vi "PV OnTool Operating adjustment.vi"(8 "error in (no error)":errorcluster, 9 "PV OnTool Op adjustment - Cluster":T1={"Parameter"=0, "Parameter\nread only<->describe"=FALSE, "off<->on"=TRUE, "Rotation speed set value\nin rot. speed setting\noperations [%]"=100.0, "Operations mode pump"=0} {"Operations mode pump" items=[" Rotations speed", " Final Speed operation", " Loadlock (Softpumping)", " Idle"]; "Rotation speed set value\nin rot. speed setting\noperations [%]" min=15.0 max=100.0 step=0.1 format="%.2f"; "Parameter" items=[" Pumping station", " Operations mode pump", " Rotation speed set value in rot. speed setting operations", " Set rotation speed BkP [Hz] (read only)", " Actual rotation speed BkP [Hz] (read only)", " Power supply version"]}, 10 "Adress of unit":u16=1 min=1 max=999 step=1, 11 "VISA session":refnum<visa-resource-name>) -> (0 "error out":errorcluster, 2 "response (data)":string, 3 "dup VISA session":refnum<visa-resource-name>)   [LabVIEW 2021, in "Pfeiffer Vacuum.lvlib"]
doc: "There are six parameters available, only one of which can be enabled at a time. \n\n0 - Pumping station [off/on] (default) (Para.010)\n1 - Operations mode pump (Para.025)\n2 - Rotation speed set value in rot. speed setting operations (Para.707)\n3 - Set rotation speed BkP [Hz] (read only) (Para.308)\n4 - Actual rotation speed BkP [Hz] (read only) (Para.309)\n5 - Power supply version (default :1 phases) (Para.029)\n\nNote: The three controls right of this one will set the appropriate values for the selected parameter. Any settings for an parameter that is not selected will be ignored. If a value is out of range, it will be changed to either the upper or the lower limit of the range."
uses:
  <instrlib>/Pfeiffer Vacuum/Pfeiffer Vacuum.lvlib
  <instrlib>/Pfeiffer Vacuum/Public/OnTool/PV OnTool Op adjustment - Cluster.ctl
panel:
  # "Pumping station                   :\n Power supply version         :"
  # "<----------\n off\n 3 phases"
  # "---------->     \non \n1 phases"
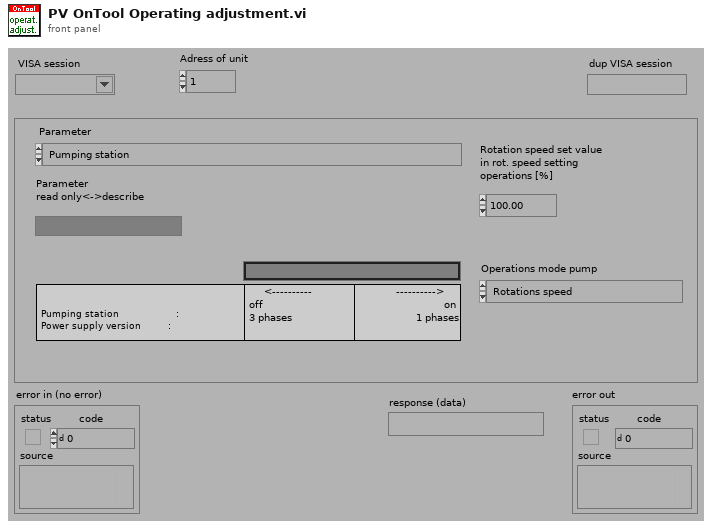
[diagram p1: front panel]
types:
  T1 = typedef "Pfeiffer Vacuum.lvlib/PV OnTool Op adjustment - Cluster.ctl" = cluster{"Parameter":u16, "Parameter\nread only<->describe":bool, "off<->on":bool, "Rotation speed set value\nin rot. speed setting\noperations [%]":dbl, "Operations mode pump":u16}
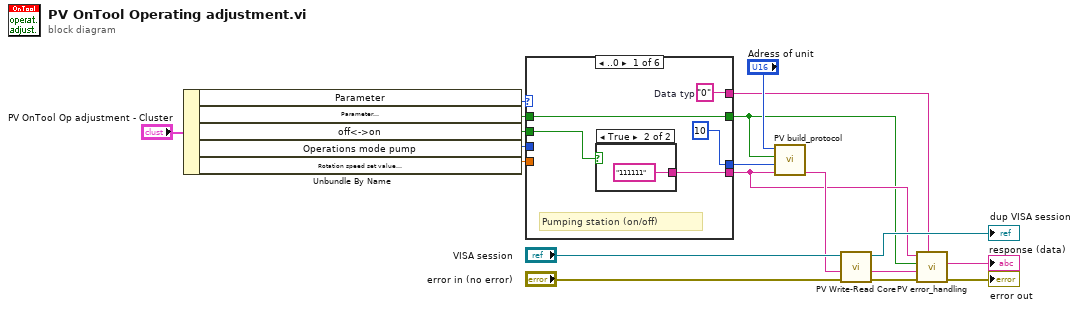
[diagram p0: block diagram]
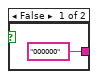
[diagram p2: hidden frame]
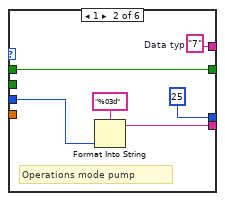
[diagram p3: hidden frame]
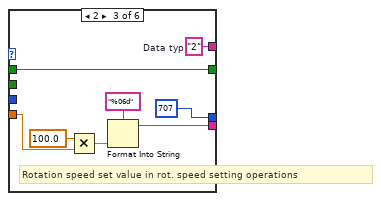
[diagram p4: hidden frame]
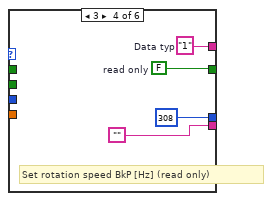
[diagram p5: hidden frame]
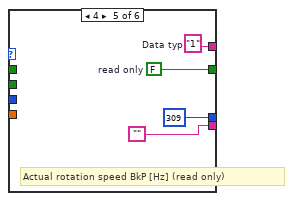
[diagram p6: hidden frame]
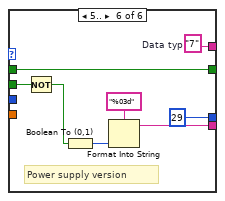
[diagram p7: hidden frame]
diagram:
  n1 = Unbundle By Name("PV OnTool Op adjustment - Cluster") -> ("Parameter"=w16:u16, "Parameter\nread only<->describe"=w15:bool, "off<->on"=w14:bool, "Operations mode pump"=w13:u16, "Rotation speed set value\nin rot. speed setting\noperations [%]"=w12:dbl)
  n2 = case shown="..0" w16 {
    tunnel: [u16 10 ("Parameter-number") u16 25 ("Parameter-number") u16 707 ("Parameter-number") u16 308 ("Parameter-number") u16 309 ("Parameter-number") u16 29 ("Parameter-number")] -> w18
    tunnel: [w23 w30 w39 "" "" w51] -> w4
    tunnel: [w22 w32 w37 w43 w47 w54] -> w3
    tunnel: w15 -> [w22 w32 w37 _ _ w54]
    tunnel: w14 -> [w21 _ _ _ _ w50]
    tunnel: w13 -> [_ w28 _ _ _ _]
    tunnel: w12 -> [_ _ w34 _ _ _]
    tunnel: [w20 w27 w33 w41 w45 w55] -> w5
    frame ..0 {
      w20 = "0"  # Data typ
      # "Pumping station (on/off)"
      n3 = case shown="True" w21 {
        tunnel: ["000000" ("Data") "111111" ("Data")] -> w23
        frame False {
        }
        frame True {
        }
      }
    }
    frame 1 {
      w27 = "7"  # Data typ
      # "Operations mode pump"
      n4 = Format Into String(format string="%03d" ("Format-String"), w28) -> (resulting string=w30:string)  [unwired: 2 in, 1 out]
    }
    frame 2 {
      w33 = "2"  # Data typ
      # "Rotation speed set value in rot. speed setting operations"
      n5 = Multiply(x=100.0, y=w34) -> (x*y=w36:dbl)
      n6 = Format Into String(format string="%06d" ("Format-String"), w36) -> (resulting string=w39:string)  [unwired: 2 in, 1 out]
    }
    frame 3 {
      w41 = "1"  # Data typ
      w43 = FALSE  # read only
      # "Set rotation speed BkP [Hz] (read only)"
    }
    frame 4 {
      w45 = "1"  # Data typ
      w47 = FALSE  # read only
      # "Actual rotation speed BkP [Hz] (read only)"
    }
    frame 5.. {
      w55 = "7"  # Data typ
      # "Power supply version"
      n7 = Not(x=w50) -> (.not. x?=w49:bool)
      n8 = Boolean To (0,1)(Boolean=w49) -> (0, 1=w52:i16)
      n9 = Format Into String(format string="%03d" ("Format-String"), w52) -> (resulting string=w51:string)  [unwired: 2 in, 1 out]
    }
  }
  n10 = call <instrlib>:"PV build_protocol.vi"("Data"=w4, "Parameter-number"=w18, "parameter\nread<->describe"=w3, "Adress"="Adress of unit") -> ("output"=w9:string)  [unwired: 3 in]
  n11 = call <instrlib>:"PV Write-Read Core.vi"("error in"="error in (no error)", "Write data in"=w9, "VISA session"="VISA session") -> ("error out"=w6:errorcluster, "response (data) out"=w7:string, "dup VISA session"=→"dup VISA session":refnum<visa-resource-name>)  [unwired: 2 in]
  n12 = call <instrlib>:"PV error_handling.vi"("Data Typ in"=w5, "error in"=w6, "response (data) in"=w7, "Parameter\nread only<->describe"=w3, "data in"=w4) -> ("error out"=→"error out":errorcluster, "Data out"=→"response (data)":string)  [unwired: 4 in, 1 out]
